vi "Close.vi"(8 "error in (no error)":errorcluster, 11 "CSV Test Log in":refnum<class "CSV Test Log.lvclass">) -> (0 "error out":errorcluster, 3 "CSV Test Log out":refnum<class "CSV Test Log.lvclass">)   [LabVIEW 2015, in "CSV Test Log.lvclass"]
uses:
  CSV Test Log.lvclass
  CSV Test Log.lvclass/CSV Test Log.ctl
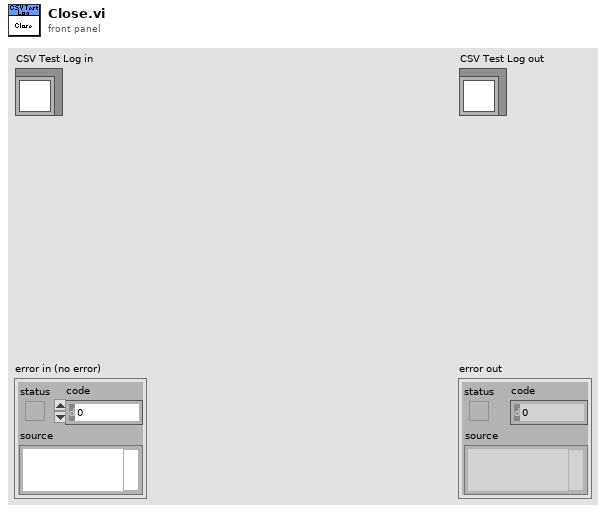
[diagram p1: front panel]
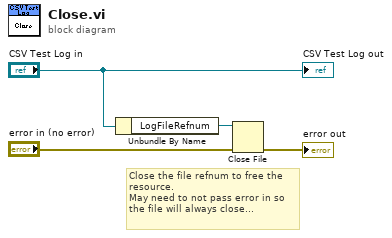
[diagram p0: block diagram]
diagram:
  # "Close the file refnum to free the\nresource.\nMay need to not pass error in so\nthe file will always close..."
  n1 = Unbundle By Name("CSV Test Log in") -> ("LogFileRefnum"=w1:refnum<file>)
  n2 = Close File(refnum=w1, error in="error in (no error)") -> (error out=→"error out":errorcluster)  [unwired: 1 out]
  "CSV Test Log out" <- "CSV Test Log in"
